vi "Teleop.vi"(10 "Match Info":T1={"Autonomous Elapsed Seconds"=0.0, "TeleOp Elapsed Seconds"=0.0, "Disabled Elapsed Seconds"=0.0, "Visited Autonomous"=FALSE, "Visited TeleOp"=FALSE, "Visited Disabled"=FALSE, "Autonomous Settings"={"Autonomous Style"=enum."Independent", "VI Refnum"=refnum}}, 11 "Call Context":T2) -> ()   [LabVIEW 2019]
doc: "This VI is called for each TeleOp packet received from the DS where the robot is not disabled. It is often used to read from the joysticks and update I/O or to update setpoints for timed control loops. It should complete and return within 20 milliseconds or it may miss DS packets."
uses:
  <vilib>/Rock Robotics/WPI/DriverStation/WPI_DriverStationDerivedRobotMode.ctl
  <vilib>/Rock Robotics/WPI/DriverStation/WPI_DriverStationMatch Info.ctl
  <vilib>/Rock Robotics/Network Tables/NT Read Boolean.vi
  <vilib>/Rock Robotics/Network Tables/NT Read Number.vi
  Global Vars.vi
  GlobalRefnum.vi
  <vilib>/Rock Robotics/WPI/Utilities/WPI_GetSetVariantRefNum.vi
  Joystick_Buttons.vi
  <vilib>/Rock Robotics/Network Tables/NT Write Boolean Array.vi
  <vilib>/Rock Robotics/Network Tables/NT Write Numeric Array.vi
  <vilib>/Rock Robotics/Network Tables/NT Write Number.vi
  <vilib>/Rock Robotics/Network Tables/NT Write Boolean.vi
panel:
  out "Shooter Side Forward?":bool
  out "left-RightArrayBR":bool
  out "left-RightArrayBM":bool
  out "left-RightArrayBL":bool
  out "left-RightArrayTL":bool
  out "left-RightArrayTM":bool
  out "left-RightArrayTR":bool
  out "left-ThumbR":bool
  out "left-ThumbL":bool
  out "left-ThumbMain":bool
  out "left-Trigger":bool
  in  "DriveScale":dbl(slide)=0.7556179775280899 min=0.25 max=1.0 step=0.1 scale=0.25..1.0
  in  "Steering Scale":dbl(slide)=0.6418539325842696 min=0.25 max=1.0 step=0.1 scale=0.25..1.0
  out "Sample Slider 0":dbl(slide) scale=0.0..5.0
  out "Sample Boolean 1":bool
  out "Sample Boolean 0":bool
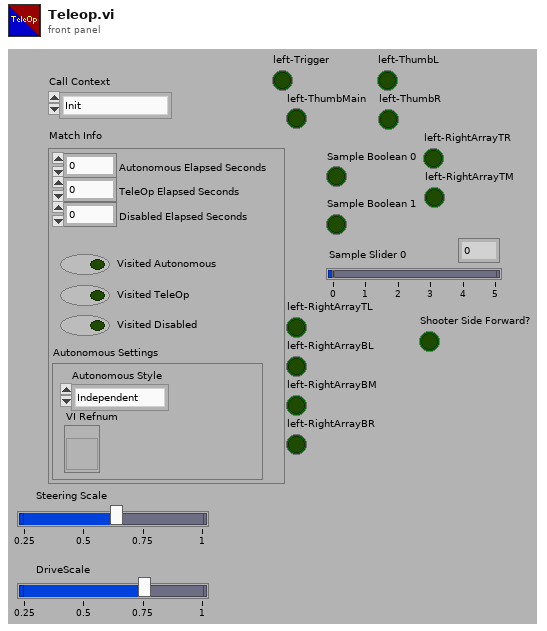
[diagram p1: front panel]
types:
  T1 = typedef "WPI_DriverStationMatch Info.ctl" = cluster{"Autonomous Elapsed Seconds":dbl, "TeleOp Elapsed Seconds":dbl, "Disabled Elapsed Seconds":dbl, "Visited Autonomous":bool, "Visited TeleOp":bool, "Visited Disabled":bool, "Autonomous Settings":cluster{"Autonomous Style":enum16{"Iterative", "Independent"}, "VI Refnum":refnum<vi>}}
  T2 = typedef "WPI_DriverStationDerivedRobotMode.ctl" = enum16{"Init", "Execute", "Stop"}
  T3 = typedef "WPI_RobotDriveDevRef.ctl" = cluster{"DevStatus":errorcluster, "Motors[]":T4[], "Square Inputs":bool, "Max Output":dbl}
  T4 = typedef "WPI_MotorControlDeviceRef.ctl" = cluster{"DeviceStatus":errorcluster, "Type":T5, "PWM":cluster{"PWM Channel":T6, "DeadBand":T7}, "CAN":cluster{"Device Number":u8, "SetOutput VI Ref":variant, "GetOutput VI Ref":variant, "Enable VI Ref":variant, "Disable VI Ref":variant, "Data":variant}, "Invert":bool, "DIO PWM":cluster{"PWM \"Enable\" Channel":T6, "DIOChannel":T8, "PWM Rate":dbl}}
  T5 = typedef "WPI_MotorControlType.ctl" = enum16{"PWM", "CAN", "DIO PWM"}
  T6 = typedef "FPGA_DIOPWMChannel.ctl" = enum8{"PWM 0", "PWM 1", "PWM 2", "PWM 3", "PWM 4", "PWM 5", "PWM 6", "PWM 7", "PWM 8", "PWM 9", "PWM MXP 0", "PWM MXP 1", "PWM MXP 2", "PWM MXP 3", "PWM MXP 4", "PWM MXP 5", "PWM MXP 6", "PWM MXP 7", "PWM MXP 8", "PWM MXP 9", "Invalid"}
  T7 = typedef "WPI_PWMDeadband.ctl" = cluster{"Name":string, "maxPositivePwm":i32, "minPositivePwm":i32, "centerPwm":i32, "maxNegativePwm":i32, "minNegativePwm":i32, "angularRange":u16}
  T8 = typedef "FPGA_DIOChannel.ctl" = enum8{"DIO 0", "DIO 1", "DIO 2", "DIO 3", "DIO 4", "DIO 5", "DIO 6", "DIO 7", "DIO 8", "DIO 9", "DIO MXP 0", "DIO MXP 1", "DIO MXP 2", "DIO MXP 3", "DIO MXP 4", "DIO MXP 5", "DIO MXP 6", "DIO MXP 7", "DIO MXP 8", "DIO MXP 9", "DIO MXP 10", "DIO MXP 11", "DIO MXP 12", "DIO MXP 13", "DIO MXP 14", "DIO MXP 15", "SPI Port CS1", "SPI Port CS2", "SPI Port CS3", "SPI Port MISO", "SPI Port MOSI", "Invalid"}
  T9 = typedef "WPI_JoystickDevRef.ctl" = cluster{"Device":T10}
  T10 = typedef "WPI_JoystickDeviceEnum.ctl" = enum16{"USB 0", "USB 1", "USB 2", "USB 3", "USB 4", "USB 5"}
  T11 = cluster{"Axes[0]":dbl, "Axes[1]":dbl, "Axes[2]":dbl, "Axes[3]":dbl, "Axes[4]":dbl, "Axes[5]":dbl, "Axes[6]":dbl, "Axes[7]":dbl, "Axes[8]":dbl}
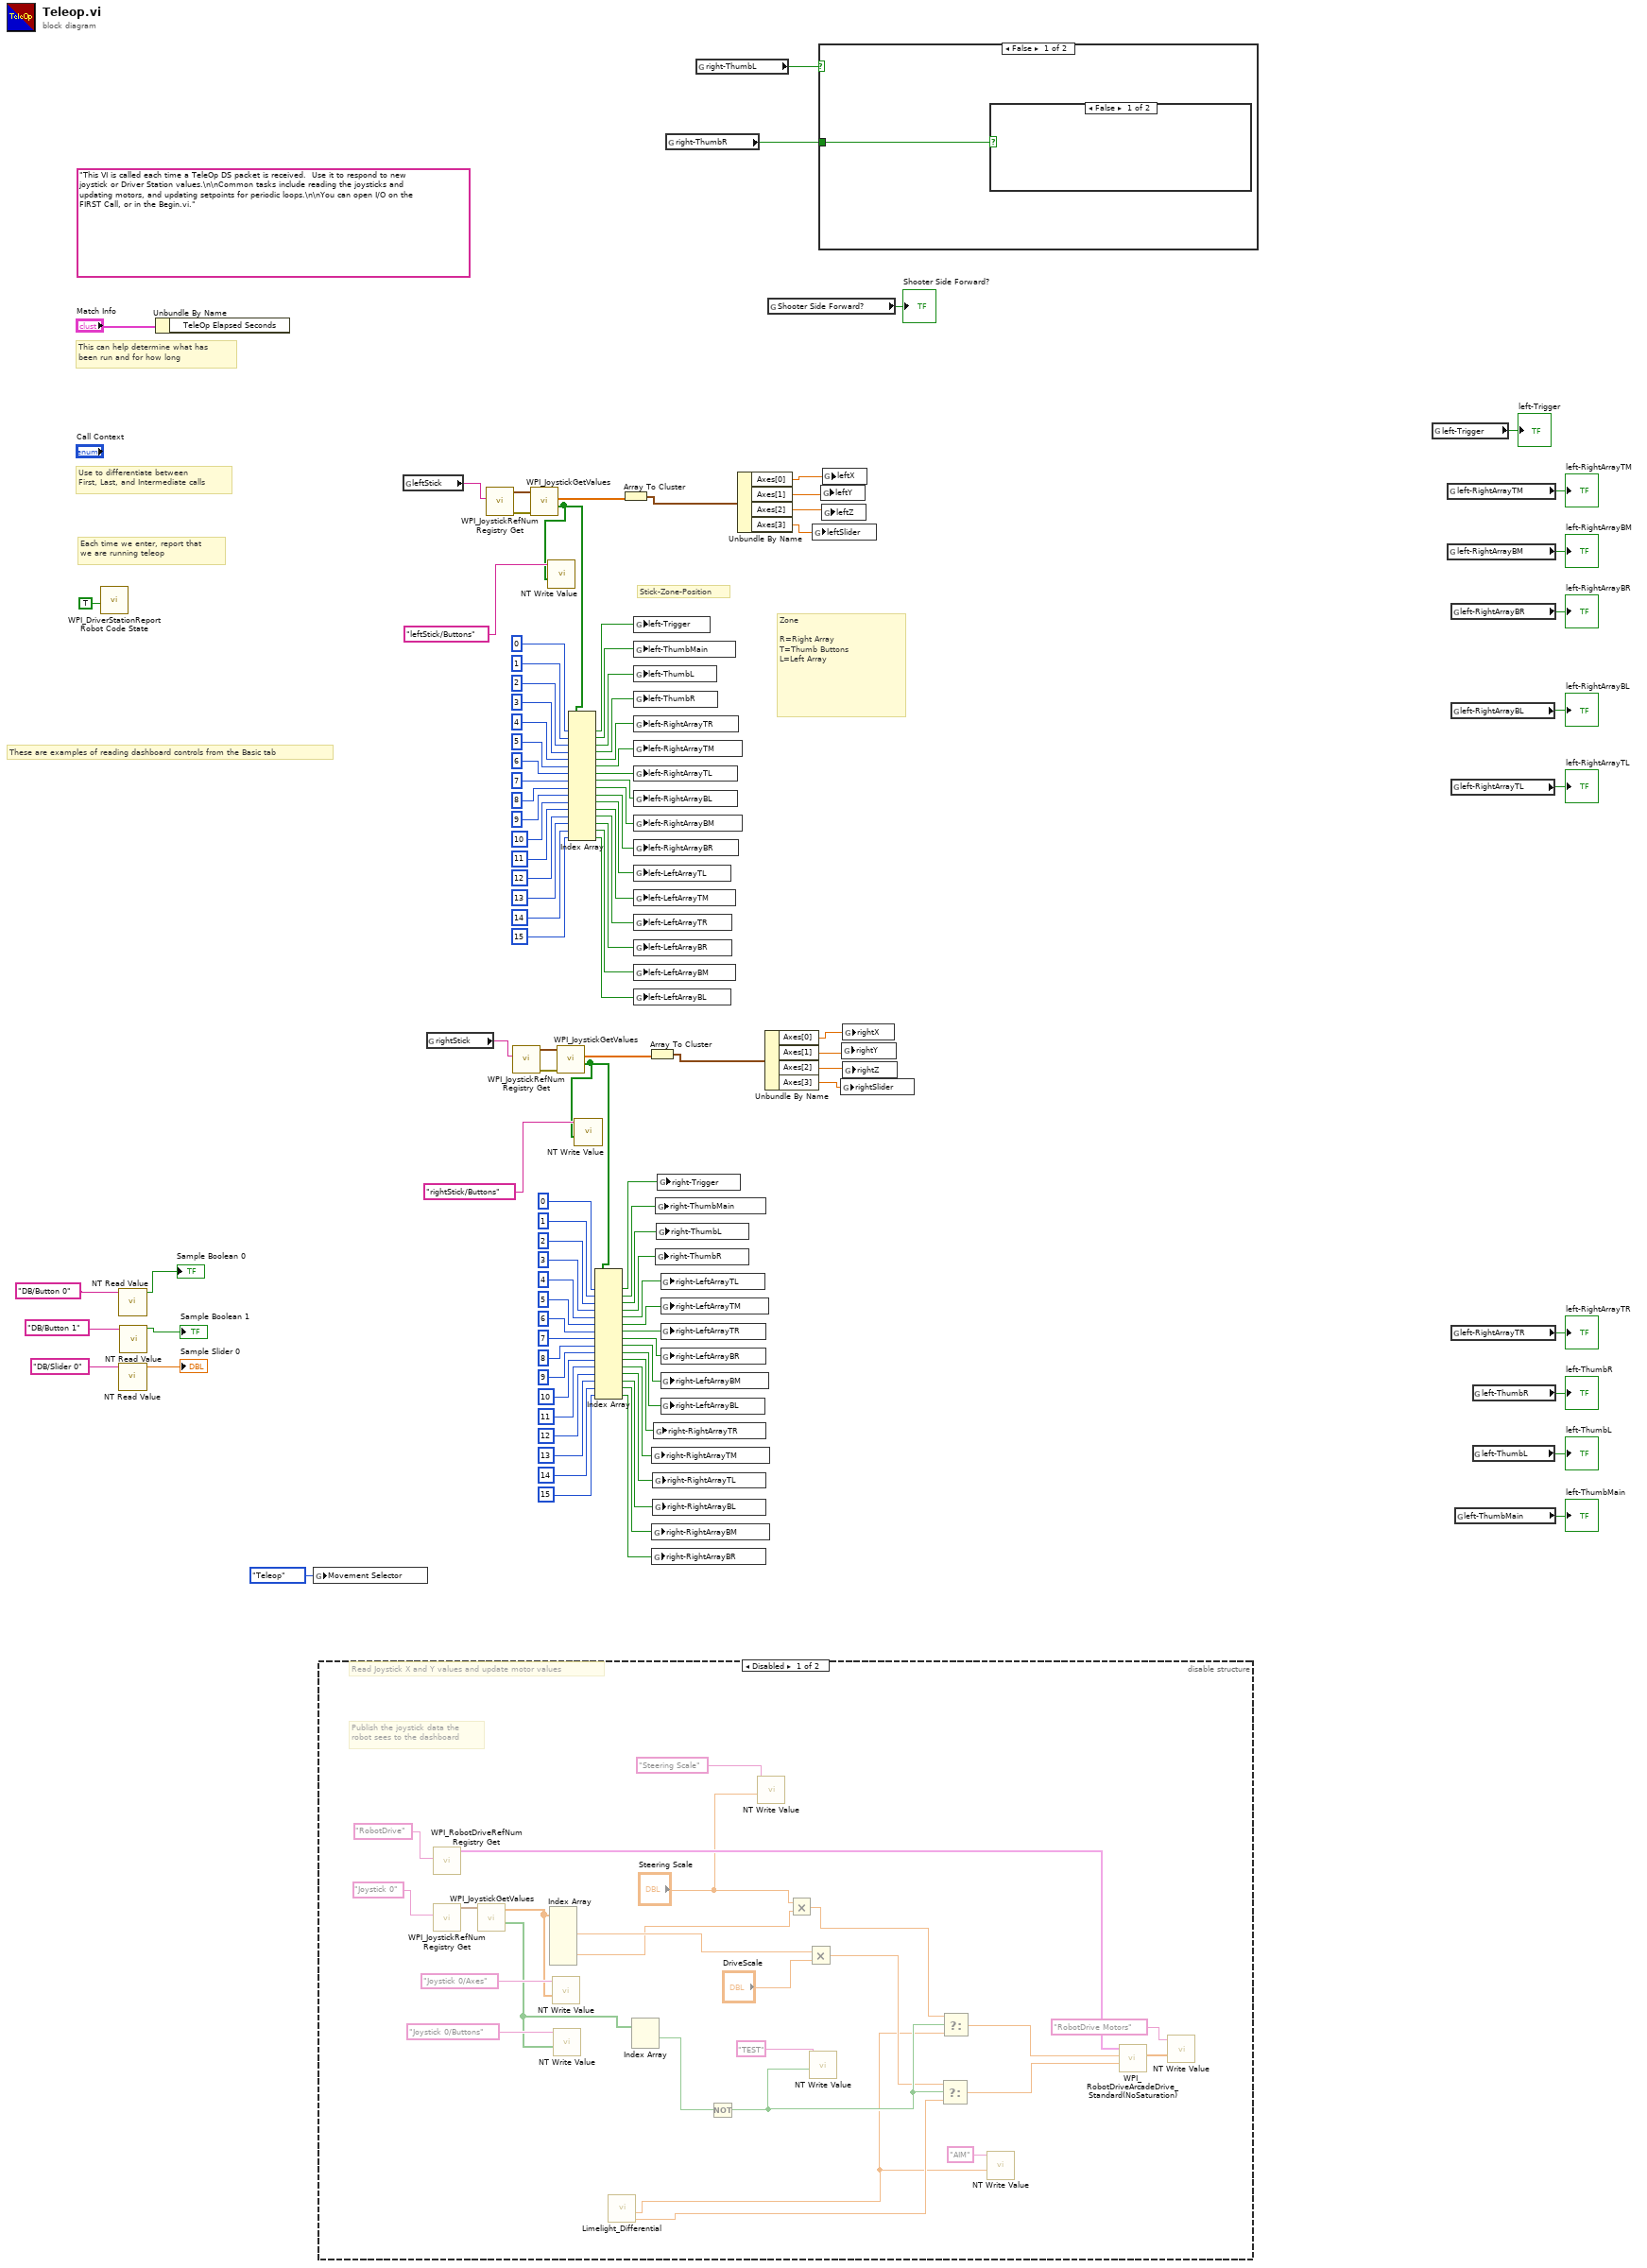
[diagram p0: block diagram]
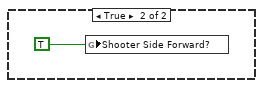
[diagram p2: hidden frame]
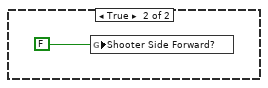
[diagram p3: hidden frame]
diagram:
  (unwired) "This VI is called each time a TeleOp DS packet is received.  Use it to respond to new joystick or Driver Station values.\n\nCommon tasks include reading the joysticks and updating motors, and updating setpoints for periodic loops.\n\nYou can open I/O on the FIRST Call, or in the Begin.vi."
  # "Zone\n\nR=Right Array\nT=Thumb Buttons\nL=Left Array"
  # "Stick-Zone-Position"
  # "These are examples of reading dashboard controls from the Basic tab"
  # "Each time we enter, report that\nwe are running teleop"
  # "Use to differentiate between\nFirst, Last, and Intermediate calls"
  # "This can help determine what has\nbeen run and for how long"
  n1 = call <vilib>:"WPI_DriverStationReport Robot Code State.vi"("TeleOp"=TRUE ("Autonomous")) -> ()  [unwired: 10 in, 1 out]
  n2 = call-poly <vilib>:"NT Read Value.vi"("Name"="DB/Button 0" ("refnum name")) -> ("Boolean"=→"Sample Boolean 0":bool)  [unwired: 9 in, 1 out]
  n3 = call-poly <vilib>:"NT Read Value.vi"("Name"="DB/Slider 0" ("refnum name")) -> ("Numeric"=→"Sample Slider 0":dbl)  [unwired: 9 in, 1 out]
  n4 = call-poly <vilib>:"NT Read Value.vi"("Name"="DB/Button 1" ("refnum name")) -> ("Boolean"=→"Sample Boolean 1":bool)  [unwired: 9 in, 1 out]
  n5 = Unbundle By Name("Match Info") -> ()  [unwired: 1 out]
  n6 = global write "Global Vars.vi" "Movement Selector"(enum16{"Teleop", "Nothin"}."Teleop" ("Movement Selector")) -> ()
  n7 = disable-structure shown="Disabled" {
    frame Disabled {
      # "Publish the joystick data the\nrobot sees to the dashboard"
      # "Read Joystick X and Y values and update motor values"
      n8 = call <vilib>:"WPI_RobotDriveRefNum Registry Get.vi"("refnum name"="RobotDrive") -> ("RobotDriveDevRef"=w132:T3)  [unwired: 1 in, 9 out]
      n9 = call <vilib>:"WPI_JoystickRefNum Registry Get.vi"("refnum name"="Joystick 0") -> ("JoystickDevRef"=w130:T9)  [unwired: 1 in, 9 out]
      n10 = call <vilib>:"WPI_JoystickGetValues.vi"("JoystickDevRef"=w130) -> ("Buttons"=w124:bool[], "Axes"=w127:dbl[])  [unwired: 6 in, 3 out]
      n11 = Index Array(array=w127) -> (element #2=w116:dbl, element #5=w111:dbl)  [unwired: 6 in, 4 out]
      n12 = call-poly <vilib>:"NT Write Value.vi"("Numeric Array"=w127, "Name"="Joystick 0/Axes") -> ()  [unwired: 9 in, 1 out]
      n13 = call-poly <vilib>:"NT Write Value.vi"("Boolean Array"=w124, "Name"="Joystick 0/Buttons") -> ()  [unwired: 9 in, 1 out]
      n14 = call "Limelight_Differential.vi"() -> ("DriveCommand"=w110:dbl, "SteerCommand"=w109:dbl)  [unwired: 8 in, 1 out]
      n15 = Index Array(array=w124) -> (element #1=w118:bool)  [unwired: 2 in, 1 out]
      n16 = Not(x=w118) -> (.not. x?=w119:bool)
      n17 = call-poly <vilib>:"NT Write Value.vi"("Numeric"="Steering Scale", "Name"="Steering Scale") -> ()  [unwired: 9 in, 1 out]
      n18 = Multiply(x="Steering Scale", y=w111) -> (x*y=w117:dbl)
      n19 = Multiply(x=w116, y="DriveScale") -> (x*y=w114:dbl)
      n20 = call-poly <vilib>:"NT Write Value.vi"("Boolean"=w119, "Name"="TEST") -> ()  [unwired: 9 in, 1 out]
      n21 = Select(t=w114, s=w119, f=w110) -> (s? t:f=w122:dbl)
      n22 = Select(t=w117, s=w119, f=w109) -> (s? t:f=w123:dbl)
      n23 = call-poly <vilib>:"NT Write Value.vi"("Numeric"=w109, "Name"="AIM") -> ()  [unwired: 9 in, 1 out]
      n24 = call <vilib>:"WPI_RobotDriveArcadeDrive_Standard(NoSaturation).vi"("Y axis value"=w122, "X axis value"=w123, "RobotDriveDevRef"=w132) -> ("Motor Values"=w126:dbl[])  [unwired: 1 in, 7 out]
      n25 = call-poly <vilib>:"NT Write Value.vi"("Numeric Array"=w126, "Name"="RobotDrive Motors") -> ()  [unwired: 9 in, 1 out]
    }
    frame Enabled {
    }
  }
  n26 = global read "GlobalRefnum.vi" "leftStick"() -> (w98:string)
  n27 = global read "GlobalRefnum.vi" "rightStick"() -> (w46:string)
  n28 = call <vilib>:"WPI_JoystickRefNum Registry Get.vi"("refnum name"=w98) -> ("error out"=w95:errorcluster, "JoystickDevRef"=w107:T9)  [unwired: 1 in, 8 out]
  n29 = call <vilib>:"WPI_JoystickRefNum Registry Get.vi"("refnum name"=w46) -> ("error out"=w43:errorcluster, "JoystickDevRef"=w48:T9)  [unwired: 1 in, 8 out]
  n30 = call <vilib>:"WPI_JoystickGetValues.vi"("error in (no error)"=w95, "JoystickDevRef"=w107) -> ("Buttons"=w91:bool[], "Axes"=w97:dbl[])  [unwired: 5 in, 3 out]
  n31 = call-poly <vilib>:"NT Write Value.vi"("Boolean Array"=w91, "Name"="leftStick/Buttons") -> ()  [unwired: 9 in, 1 out]
  n32 = call <vilib>:"WPI_JoystickGetValues.vi"("error in (no error)"=w43, "JoystickDevRef"=w48) -> ("Buttons"=w40:bool[], "Axes"=w45:dbl[])  [unwired: 5 in, 3 out]
  n33 = Index Array(array=w91, index #1=0 ("index"), index #2=1 ("index"), index #3=2 ("index"), index #4=3 ("index"), index #5=4 ("index"), index #6=5 ("index"), index #7=6 ("index"), index #8=7 ("index"), index #9=8 ("index"), index #10=9 ("index"), index #11=10 ("index"), index #12=11 ("index"), index #13=12 ("index"), index #14=13 ("index"), index #15=14 ("index"), index #16=15 ("index")) -> (element #1=w80:bool, element #2=w79:bool, element #3=w78:bool, element #4=w77:bool, element #5=w76:bool, element #6=w75:bool, element #7=w74:bool, element #8=w73:bool, element #9=w72:bool, element #10=w71:bool, element #11=w54:bool, element #12=w53:bool, element #13=w52:bool, element #14=w51:bool, element #15=w50:bool, element #16=w49:bool)
  n34 = call-poly <vilib>:"NT Write Value.vi"("Boolean Array"=w40, "Name"="rightStick/Buttons") -> ()  [unwired: 9 in, 1 out]
  n35 = Index Array(array=w40, index #1=0 ("index"), index #2=1 ("index"), index #3=2 ("index"), index #4=3 ("index"), index #5=4 ("index"), index #6=5 ("index"), index #7=6 ("index"), index #8=7 ("index"), index #9=8 ("index"), index #10=9 ("index"), index #11=10 ("index"), index #12=11 ("index"), index #13=12 ("index"), index #14=13 ("index"), index #15=14 ("index"), index #16=15 ("index")) -> (element #1=w29:bool, element #2=w28:bool, element #3=w27:bool, element #4=w26:bool, element #5=w25:bool, element #6=w24:bool, element #7=w23:bool, element #8=w22:bool, element #9=w21:bool, element #10=w20:bool, element #11=w13:bool, element #12=w12:bool, element #13=w11:bool, element #14=w10:bool, element #15=w9:bool, element #16=w8:bool)
  n36 = Array To Cluster(array=w97) -> (cluster=w96:T11)
  n37 = global write "Joystick_Buttons.vi" "left-Trigger"(w80) -> ()
  n38 = global write "Joystick_Buttons.vi" "left-ThumbMain"(w79) -> ()
  n39 = global write "Joystick_Buttons.vi" "left-ThumbL"(w78) -> ()
  n40 = global write "Joystick_Buttons.vi" "left-ThumbR"(w77) -> ()
  n41 = global write "Joystick_Buttons.vi" "left-RightArrayTR"(w76) -> ()
  n42 = global write "Joystick_Buttons.vi" "left-RightArrayTM"(w75) -> ()
  n43 = global write "Joystick_Buttons.vi" "left-RightArrayTL"(w74) -> ()
  n44 = global write "Joystick_Buttons.vi" "left-RightArrayBL"(w73) -> ()
  n45 = global write "Joystick_Buttons.vi" "left-RightArrayBM"(w72) -> ()
  n46 = global write "Joystick_Buttons.vi" "left-RightArrayBR"(w71) -> ()
  n47 = global write "Joystick_Buttons.vi" "left-LeftArrayTL"(w54) -> ()
  n48 = global write "Joystick_Buttons.vi" "left-LeftArrayTM"(w53) -> ()
  n49 = global write "Joystick_Buttons.vi" "left-LeftArrayTR"(w52) -> ()
  n50 = global write "Joystick_Buttons.vi" "left-LeftArrayBR"(w51) -> ()
  n51 = global write "Joystick_Buttons.vi" "left-LeftArrayBM"(w50) -> ()
  n52 = global write "Joystick_Buttons.vi" "left-LeftArrayBL"(w49) -> ()
  n53 = Array To Cluster(array=w45) -> (cluster=w44:T11)
  n54 = global write "Joystick_Buttons.vi" "right-RightArrayTM"(w12) -> ()
  n55 = global write "Joystick_Buttons.vi" "right-RightArrayBM"(w9) -> ()
  n56 = global write "Joystick_Buttons.vi" "right-RightArrayBR"(w8) -> ()
  n57 = global write "Joystick_Buttons.vi" "right-RightArrayTL"(w11) -> ()
  n58 = global write "Joystick_Buttons.vi" "right-RightArrayBL"(w10) -> ()
  n59 = global write "Joystick_Buttons.vi" "right-RightArrayTR"(w13) -> ()
  n60 = global write "Joystick_Buttons.vi" "right-ThumbMain"(w28) -> ()
  n61 = global write "Joystick_Buttons.vi" "right-ThumbR"(w26) -> ()
  n62 = global write "Joystick_Buttons.vi" "right-ThumbL"(w27) -> ()
  n63 = global write "Joystick_Buttons.vi" "right-Trigger"(w29) -> ()
  n64 = global write "Joystick_Buttons.vi" "right-LeftArrayTL"(w25) -> ()
  n65 = global write "Joystick_Buttons.vi" "right-LeftArrayTM"(w24) -> ()
  n66 = global write "Joystick_Buttons.vi" "right-LeftArrayTR"(w23) -> ()
  n67 = global write "Joystick_Buttons.vi" "right-LeftArrayBR"(w22) -> ()
  n68 = global write "Joystick_Buttons.vi" "right-LeftArrayBM"(w21) -> ()
  n69 = global write "Joystick_Buttons.vi" "right-LeftArrayBL"(w20) -> ()
  n70 = global read "Joystick_Buttons.vi" "right-ThumbR"() -> (w6:bool)
  n71 = global read "Joystick_Buttons.vi" "right-ThumbL"() -> (w5:bool)
  n72 = Unbundle By Name(w96) -> ("Axes[0]"=w94:dbl, "Axes[1]"=w93:dbl, "Axes[2]"=w92:dbl, "Axes[3]"=w2:dbl)
  n73 = Unbundle By Name(w44) -> ("Axes[0]"=w7:dbl, "Axes[1]"=w42:dbl, "Axes[2]"=w41:dbl, "Axes[3]"=w1:dbl)
  n74 = global read "Global Vars.vi" "Shooter Side Forward?"() -> (→"Shooter Side Forward?":bool)
  n75 = global write "Joystick_Buttons.vi" "leftSlider"(w2) -> ()
  n76 = case shown="False" w5 {
    tunnel: w6 -> [w134 _]
    frame False {
      n77 = case shown="False" w134 {
        frame False {
        }
        frame True {
          n78 = global write "Global Vars.vi" "Shooter Side Forward?"(TRUE ("State")) -> ()
        }
      }
    }
    frame True {
      n79 = global write "Global Vars.vi" "Shooter Side Forward?"(FALSE) -> ()
    }
  }
  n80 = global write "Joystick_Buttons.vi" "leftY"(w93) -> ()
  n81 = global write "Joystick_Buttons.vi" "leftZ"(w92) -> ()
  n82 = global write "Joystick_Buttons.vi" "leftX"(w94) -> ()
  n83 = global write "Joystick_Buttons.vi" "rightSlider"(w1) -> ()
  n84 = global write "Joystick_Buttons.vi" "rightY"(w42) -> ()
  n85 = global write "Joystick_Buttons.vi" "rightX"(w7) -> ()
  n86 = global write "Joystick_Buttons.vi" "rightZ"(w41) -> ()
  n87 = global read "Joystick_Buttons.vi" "left-Trigger"() -> (→"left-Trigger":bool)
  n88 = global read "Joystick_Buttons.vi" "left-RightArrayTM"() -> (→"left-RightArrayTM":bool)
  n89 = global read "Joystick_Buttons.vi" "left-RightArrayBM"() -> (→"left-RightArrayBM":bool)
  n90 = global read "Joystick_Buttons.vi" "left-RightArrayBR"() -> (→"left-RightArrayBR":bool)
  n91 = global read "Joystick_Buttons.vi" "left-RightArrayBL"() -> (→"left-RightArrayBL":bool)
  n92 = global read "Joystick_Buttons.vi" "left-RightArrayTL"() -> (→"left-RightArrayTL":bool)
  n93 = global read "Joystick_Buttons.vi" "left-RightArrayTR"() -> (→"left-RightArrayTR":bool)
  n94 = global read "Joystick_Buttons.vi" "left-ThumbMain"() -> (→"left-ThumbMain":bool)
  n95 = global read "Joystick_Buttons.vi" "left-ThumbR"() -> (→"left-ThumbR":bool)
  n96 = global read "Joystick_Buttons.vi" "left-ThumbL"() -> (→"left-ThumbL":bool)
